vi "Update Seq.vi"(8 "Error In":errorcluster, 9 "Sequence":T1(array[cluster])=[{"Duration"=0, "Value"=1, "Name"="Step1"}, {"Duration"=10, "Value"=2, "Name"="Step2"}, {"Duration"=10, "Value"=4, "Name"="Step3"}, {"Duration"=20, "Value"=0, "Name"="Step4"}, {"Duration"=20, "Value"=0, "Name"="Step5"}, {"Duration"=30, "Value"=0, "Name"="Step6"}, {"Duration"=30, "Value"=0, "Name"="Step7"}, {"Duration"=40, "Value"=0, "Name"="Step8"}, {"Duration"=40, "Value"=100, "Name"="Step9"}, {"Duration"=50, "Value"=0, "Name"="Step10"}], 10 "file path":path, 11 "Sequence in":refnum<class "Sequence.lvclass">) -> (0 "error out":errorcluster, 3 "Sequence out":refnum<class "Sequence.lvclass">)   [LabVIEW 2019, in "Sequence.lvlib" / "Sequence.lvclass"]
uses:
  Sequence.lvclass
  <vilib>/Utility/config.llb/Write Key (String).vi
  <vilib>/Utility/config.llb/Write Key (I32).vi
  <vilib>/Utility/config.llb/Write Key (Double).vi
  <vilib>/Utility/config.llb/NI_LVConfig.lvlib
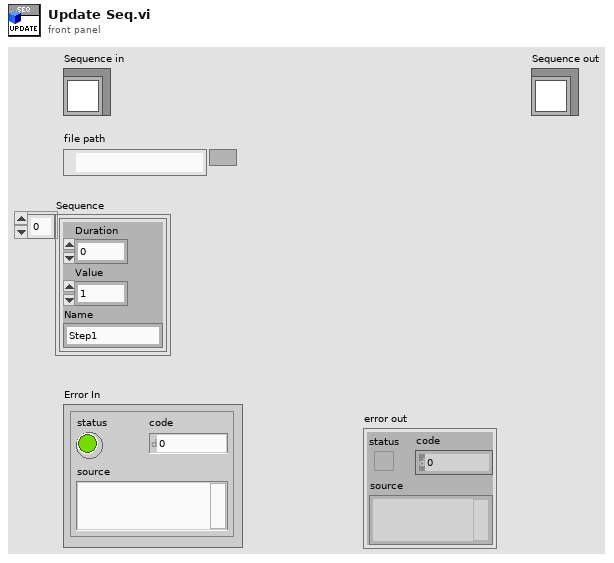
[diagram p1: front panel]
types:
  T1 = cluster{"Duration":i32, "Value":u32, "Name":string}[]
  T2 = typedef "NI_LVConfig.lvlib/Config Data RefNum.ctl" = refnum<k1>
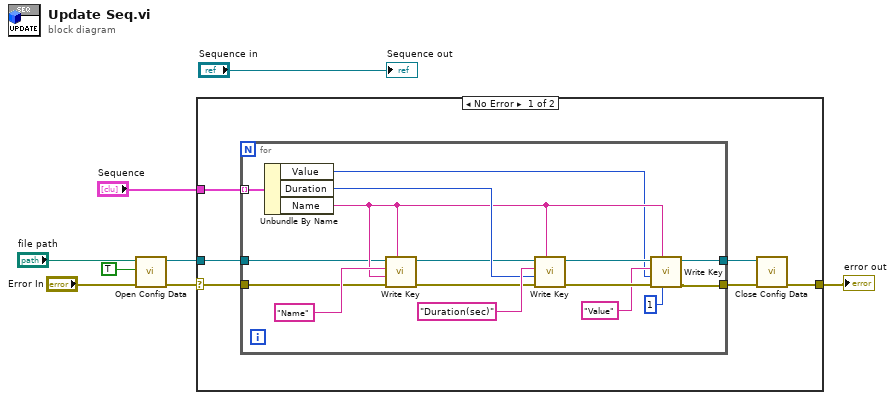
[diagram p0: block diagram]
diagram:
  n1 = call <vilib>:"Open Config Data.vi"("error in (no error)"="Error In", "create file if necessary (T)"=TRUE, "configuration file path"="file path") -> ("error out"=w4:errorcluster, "refnum"=w5:T2)  [unwired: 6 in, 1 out]
  n2 = case shown="No Error" w4 {
    selector: w4 -> [w11 w31]
    tunnel: [w14 w31] -> w8
    tunnel: w5 -> [w12 _]
    tunnel: "Sequence" -> [w9 _]
    frame No Error {
      n3 = for {
        tunnel: w9 -> [w29] mode=indexing
        tunnel: w11 -> [w20]
        tunnel: w12 -> [w19]
        tunnel: [w17] -> w13
        tunnel: [w15] -> w10
        n4 = Unbundle By Name(w29) -> ("Value"=w16:u32, "Duration"=w28:i32, "Name"=w22:string)
        n5 = call-poly <vilib>:"Write Key.vi"("section"=w22, "error in (no error)"=w20, "value"=w22, "key"="Name", "refnum"=w19) -> ("error out"=w25:errorcluster, "refnum out"=w23:T2)  [unwired: 4 in, 1 out]
        n6 = call-poly <vilib>:"Write Key.vi"("section"=w22, "error in (no error)"=w25, "value"=w28, "key"="Duration(sec)", "refnum"=w23) -> ("error out"=w27:errorcluster, "refnum out"=w26:T2)  [unwired: 4 in, 1 out]
        n7 = call-poly <vilib>:"Write Key.vi"("precision (6)"=i16 1, "section"=w22, "error in (no error)"=w27, "value"=w16, "key"="Value", "refnum"=w26) -> ("error out"=w17:errorcluster, "refnum out"=w15:T2)  [unwired: 3 in, 1 out]
      }
      n8 = call <vilib>:"Close Config Data.vi"("error in (no error)"=w13, "refnum"=w10) -> ("error out"=w14:errorcluster)  [unwired: 8 in, 1 out]
    }
    frame Error {
    }
  }
  "error out" <- w8
  "Sequence out" <- "Sequence in"
